vi "SIMPLE_Read_2_motors.vi"() -> ()   [LabVIEW 2016]
uses:
  <vilib>/Instr/_visa.llb/VISA Set IO Buffer Mask.ctl
  <vilib>/Utility/miscctls.llb/LVPointTypeDef.ctl
  <vilib>/Instr/_visa.llb/VISA Configure Serial Port (Instr).vi
  GEN_2.lvlib
  <vilib>/Analysis/NI_AALBase.lvlib
  <vilib>/Analysis/NI_AALPro.lvlib
  <vilib>/Analysis/baseanly.llb/Mean (DBL).vi
  GEN2_Stat_Addr.ctl
panel:
  out "Error_count":dbl[](array[numeric])
  in  "Array":u8[](array[numeric]) format="%x"
  out "Histogram":T1(graph)
  in  "stop 2":bool
  out "mean_hz":dbl format="%0.2f"
  out "Waveform Chart":dbl(graph)
  in  "Address":T2[](array[typedef])=[9, 10, 11, 12, 13] items=["Torque Enable", "Homing Complete", "Goal Id", "Goal Iq", "Goal Velo", "Goal Posi", "Present Id", "Present Iq", "Present Velo", "Present Posi", "Bus Voltage", "Temperature Winding", "Temperature MOSFET", "Temperature IC", "Error Status", "Iq_Temps"]
  out "ERROR":u8
  out "value":dbl[](array[numeric])=[2903.94775390625, 24.112640380859375, 25.25, 24.875, 27.875]
  in  "read":bool
  in  "Baud rate":u32=8000000
  in  "Com port":refnum<visa-resource-name>="COM8"
  in  "stop":bool
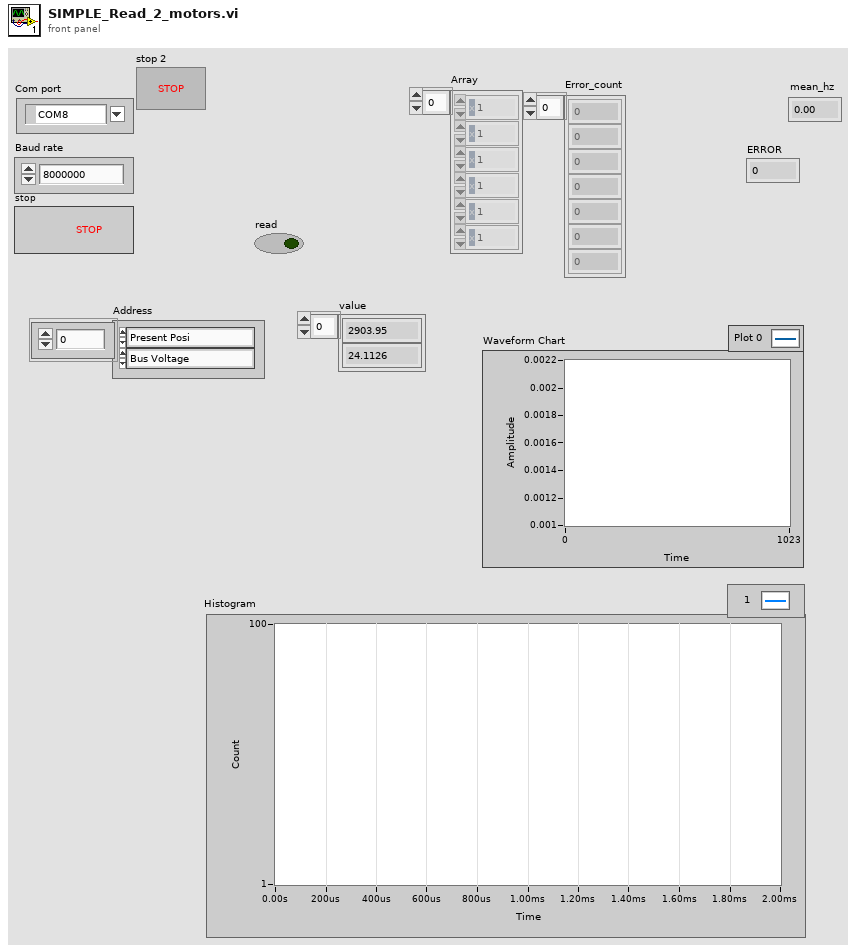
[diagram p1: front panel]
types:
  T1 = cluster{"X Values":dbl[], "Histogram: h(x)":i32[]}
  T2 = typedef "GEN_2.lvlib/GEN2_Stat_Addr.ctl" = u8
  T3 = typedef "LVPointTypeDef.ctl" = cluster{"Horizontal":i16, "Vertical":i16}
  T4 = typedef "VISA Set IO Buffer Mask.ctl" = u16
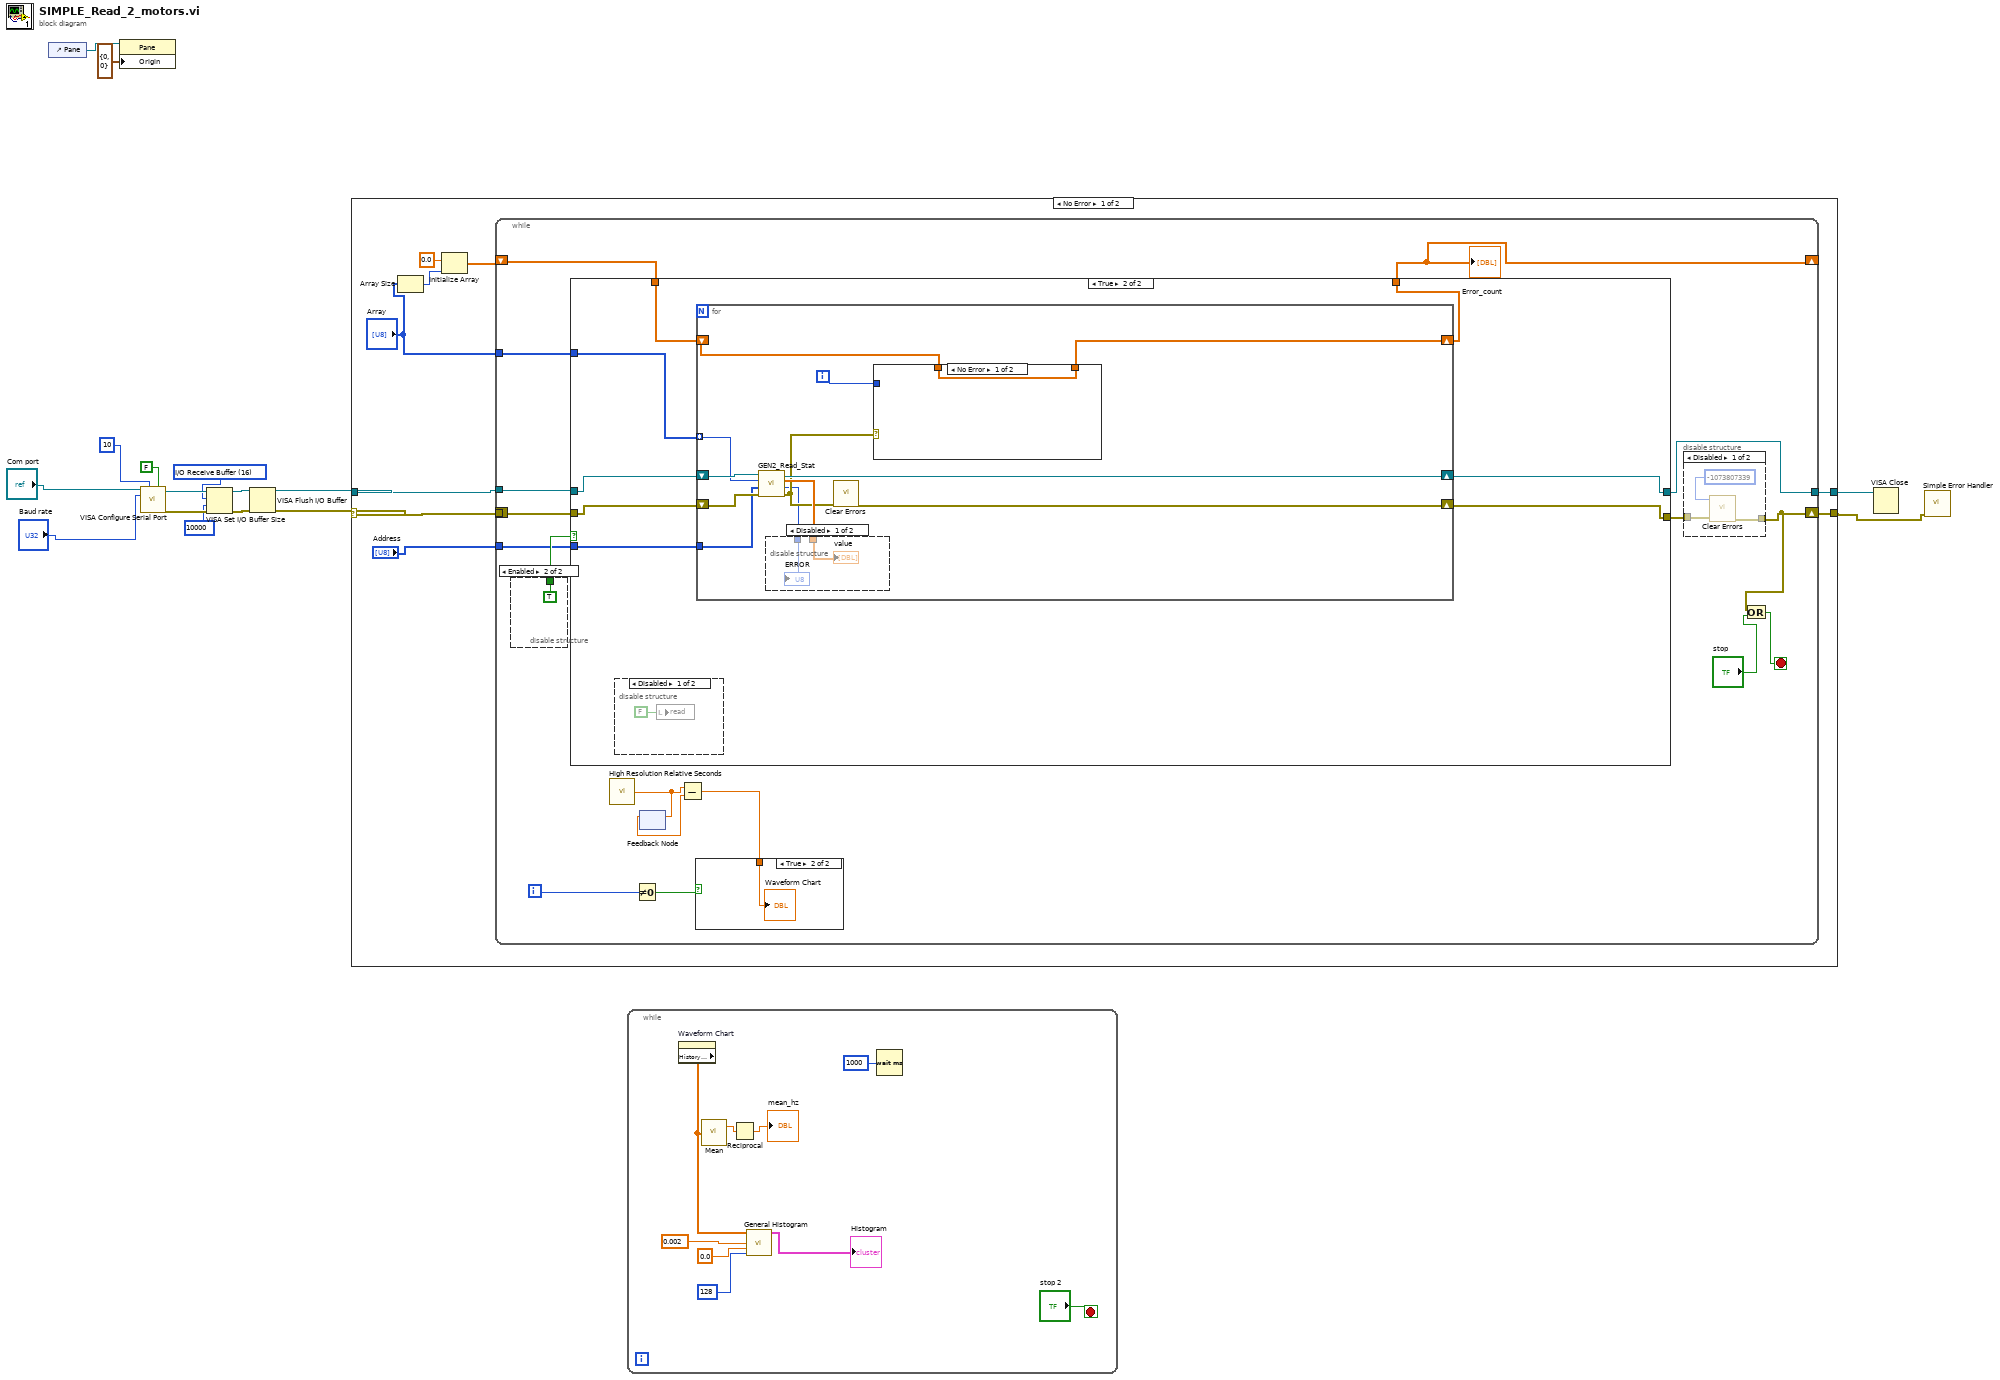
[diagram p0: block diagram]
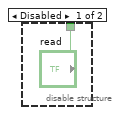
[diagram p2: hidden frame]
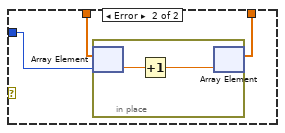
[diagram p7: hidden frame]
diagram:
  w9 = T4 16 items=["I/O Receive Buffer"=16, "I/O Transmit Buffer"=32, "I/O Receive and Transmit Buffer"=48] ("Mask")
  n1 = control-ref of="Pane"() -> (w5:refnum<vi>)
  n2 = property class="Pane"(reference=w5, "Origin"=T3 {"Horizontal"=0, "Vertical"=0}) -> ()  [unwired: 1 in, 2 out]
  n3 = call-poly "VISA Configure Serial Port"("VISA resource name"="Com port", "timeout (10sec)"=u32 10, "Enable Termination\nChar (T)"=FALSE ("Enable Termination\nChar (T)"), "baud rate (9600)"="Baud rate") -> ("VISA resource name out"=w10:refnum<visa-resource-name>, "error out"=w13:errorcluster)  [unwired: 10 in]
  n4 = VISA Set I/O Buffer Size(VISA resource name=w10, mask (16)=w9, size (4096)=u32 10000, error in (no error)=w13) -> (VISA resource name out=w11:refnum<visa-resource-name>, error out=w12:errorcluster)
  n5 = VISA Flush I/O Buffer(VISA resource name=w11, error in (no error)=w12) -> (VISA resource name out=w2:refnum<visa-resource-name>, error out=w3:errorcluster)  [unwired: 1 in]
  n6 = case shown="No Error" w3 {
    selector: w3 -> [w22 w82]
    tunnel: [w25 w82] -> w1
    tunnel: w2 -> [w24 w83]
    tunnel: [w23 w83] -> w15
    frame No Error {
      n7 = Array Size(array="Array") -> (size(s)=w19:i32)
      n8 = Initialize Array(0.0 ("element"), w19) -> (w17:dbl[])
      n9 = while {
        tunnel: w24 -> [w39]
        tunnel: w22 -> [w38]
        tunnel: [w36] -> w23
        shift-right: [w37] -> w25
        shift-left: _ -> [_]
        tunnel: "Array" -> [w29]
        tunnel: "Address" -> [w28]
        shift-right: [w26] -> _
        shift-left: w17 -> [w27]
        i -> [w34]
        stop <- w41 stop-if-true
        n10 = disable-structure shown="Enabled" {
          disable-tunnel: ["read" TRUE ("read")] -> w40
          frame Disabled {
          }
          frame Enabled {
          }
        }
        n11 = case shown="True" w40 {
          tunnel: w38 -> [w52 w60]
          tunnel: w39 -> [w51 w59]
          tunnel: [w51 w57] -> w36
          tunnel: [w52 w58] -> w35
          tunnel: w29 -> [_ w56]
          tunnel: w28 -> [_ w55]
          tunnel: w27 -> [w50 w54]
          tunnel: [w50 w53] -> w26
          frame False {
          }
          frame True {
            n12 = disable-structure shown="Disabled" {
              frame Disabled {
                n13 = local write "read"(FALSE ("write")) -> ()
              }
              frame Enabled {
              }
            }
            n14 = for {
              tunnel: w56 -> [w70] mode=indexing
              tunnel: w55 -> [w65]
              shift-right: [w66] -> w58
              shift-left: w60 -> [w72]
              shift-right: [w69] -> w57
              shift-left: w59 -> [w71]
              shift-right: [w61] -> w53
              shift-left: w54 -> [w63]
              i -> [w62]
              n15 = call "GEN2_Read_Stat.vi"("error in (no error)"=w72, "Stat Address"=w65, "ID"=w70, "VISA Refnum in"=w71) -> ("error out"=w67:errorcluster, "ERROR"=w64:u8, "Data"=w68:dbl[], "VISA Refnum out"=w69:refnum<visa-resource-name>)  [unwired: 4 in]
              n16 = disable-structure shown="Disabled" {
                disable-tunnel: w68 -> [w74 _]
                disable-tunnel: w64 -> [w73 _]
                frame Disabled {
                  "value" <- w74
                  "ERROR" <- w73
                }
                frame Enabled {
                }
              }
              n17 = call <vilib>:"Clear Errors.vi"("error in (no error)"=w67) -> ("error out"=w66:errorcluster)  [unwired: 5 in, 1 out]
              n18 = case shown="No Error" w67 {
                tunnel: w63 -> [w75 w78]
                tunnel: w62 -> [_ w77]
                tunnel: [w75 w76] -> w61
                frame No Error {
                }
                frame Error {
                  n19 = in-place {
                    n20 = in-place-array #1(w78, w77) -> (w80:dbl)
                    n21 = Increment(x=w80) -> (x+1=w79:dbl)
                    n22 = in-place-array #1(w79) -> (w76:dbl[])  [unwired: 1 out]
                  }
                }
              }
            }
          }
        }
        "Error_count" <- w26
        n23 = call <vilib>:"High Resolution Relative Seconds.vi"() -> ("relative seconds"=w31:dbl)
        n24 = Not Equal To 0?(x=w34) -> (x != 0?=w33:bool)
        n25 = feedback #2() -> (w32:dbl)  [unwired: 1 in]
        n26 = feedback-in #2(w31) -> ()
        n27 = Subtract(x=w31, y=w32) -> (x-y=w30:dbl)
        n28 = case shown="True" w33 {
          tunnel: w30 -> [_ w45]
          frame False {
          }
          frame True {
            "Waveform Chart" <- w45
          }
        }
        n29 = disable-structure shown="Disabled" {
          disable-tunnel: [w47 w49] -> w37
          disable-tunnel: w35 -> [w46 w49]
          frame Disabled {
            n30 = call <vilib>:"Clear Errors.vi"("error in (no error)"=w46, "specific error code to clear (0: all)"=-1073807339) -> ("error out"=w47:errorcluster)  [unwired: 4 in, 1 out]
          }
          frame Enabled {
          }
        }
        n31 = Or(x=w37, y="stop") -> (x .or. y?=w41:bool)
      }
    }
    frame Error {
    }
  }
  n32 = while {
    stop <- "stop 2" stop-if-true
    n33 = property on="Waveform Chart" class="WFChart (strict)"() -> ("History Data"=w90:dbl[])  [unwired: 2 in, 2 out]
    n34 = call-poly <vilib>:"Mean.vi"("X"=w90) -> ("mean"=w87:dbl)  [unwired: 1 out]
    n35 = Reciprocal(x=w87) -> (1/x=→"mean_hz":dbl)
    n36 = call <vilib>:"General Histogram.vi"("X"=w90, "max"=0.002, "min"=0.0, "# bins"=128) -> ("Histogram Graph"=→"Histogram":T1)  [unwired: 7 in, 4 out]
    n37 = Wait (ms)(milliseconds to wait=u32 1000) -> ()  [unwired: 1 out]
  }
  n38 = VISA Close(VISA resource name=w15) -> ()  [unwired: 1 in, 1 out]
  n39 = call <vilib>:"Simple Error Handler.vi"("error in (no error)"=w1) -> ()  [unwired: 4 in, 5 out]
